vi "SonarsUpdate.vi"() -> ()   [LabVIEW 2016]
uses:
  <vilib>/Rock Robotics/WPI/Ultrasonic/WPI_UltrasonicRangeUnits.ctl
  <vilib>/Rock Robotics/WPI/Ultrasonic/WPI_SonarSRF04DigitalRefNum Registry Get.vi
  <vilib>/Rock Robotics/WPI/Ultrasonic/WPI_SonarSRF04DigitalGetRange.vi
  Globals/Globals.vi
  <vilib>/Rock Robotics/Network Tables/NT Write Number.vi
panel:
  in  "Sensor Droite Enable":bool
  in  "Sensor Gauche Enable":bool
  out "Waveform G":dbl(graph)
  out "Sensor Gauche":dbl
  out "Waveform  D":dbl(graph)
  out "Sensor Droite":dbl
  in  "Sensors Ping Duration (s)":sgl=1e-05
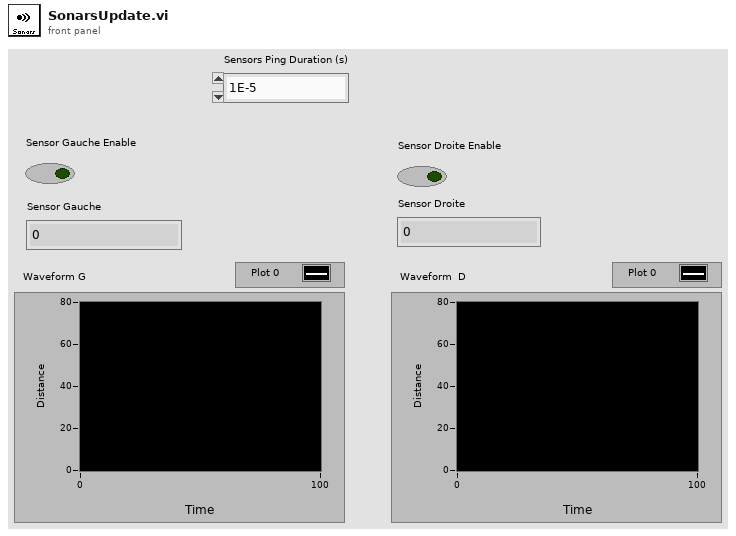
[diagram p1: front panel]
types:
  T1 = typedef "WPI_UltrasonicRangeUnits.ctl" = enum16{"inches", "mm"}
  T2 = typedef "WPI_UltrasonicDeviceRef.ctl" = cluster{"DevStatus":errorcluster, "Ping Channel":T3, "Echo Channel":T3, "CntIndex":T4}
  T3 = typedef "FPGA_DIOChannel.ctl" = enum8{"DIO 0", "DIO 1", "DIO 2", "DIO 3", "DIO 4", "DIO 5", "DIO 6", "DIO 7", "DIO 8", "DIO 9", "DIO MXP 0", "DIO MXP 1", "DIO MXP 2", "DIO MXP 3", "DIO MXP 4", "DIO MXP 5", "DIO MXP 6", "DIO MXP 7", "DIO MXP 8", "DIO MXP 9", "DIO MXP 10", "DIO MXP 11", "DIO MXP 12", "DIO MXP 13", "DIO MXP 14", "DIO MXP 15", "SPI Port CS1", "SPI Port CS2", "SPI Port CS3", "SPI Port MISO", "SPI Port MOSI", "Invalid"}
  T4 = typedef "FPGA_CounterCtrSystemIndex.ctl" = enum8{"Ctr 0", "Ctr 1", "Ctr 2", "Ctr 3", "Ctr 4", "Ctr 5", "Ctr 6", "Ctr 7", "Invalid"}
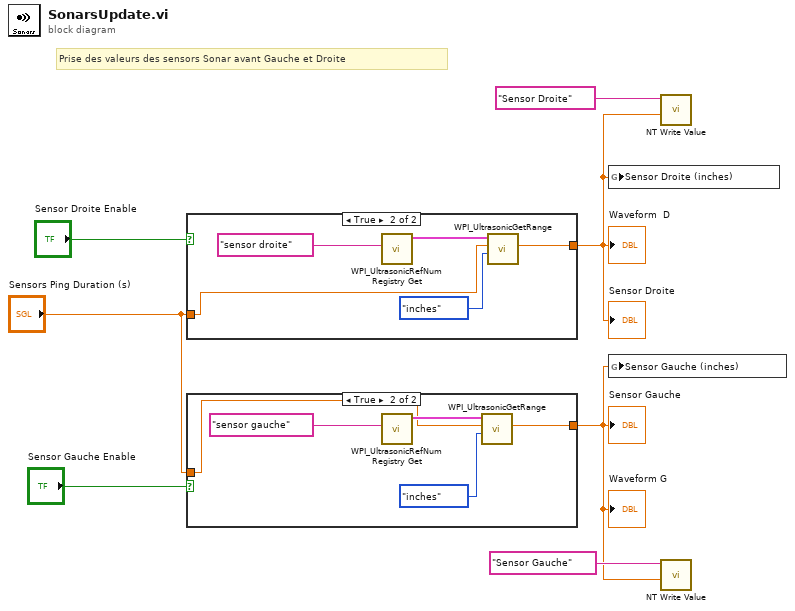
[diagram p0: block diagram]
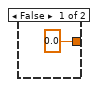
[diagram p2: hidden frame]
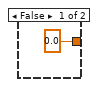
[diagram p3: hidden frame]
diagram:
  # "Prise des valeurs des sensors Sonar avant Gauche et Droite"
  n1 = case shown="True" "Sensor Droite Enable" {
    tunnel: "Sensors Ping Duration (s)" -> [_ w10]
    tunnel: [0.0 ("Distance") w9] -> w5
    frame False {
    }
    frame True {
      n2 = call-poly <vilib>:"WPI_UltrasonicRefNum Registry Get.vi"("refnum name"="sensor droite") -> ("SonarSRF04DevRef"=w13:T2)  [unwired: 9 in, 1 out]
      n3 = call-poly <vilib>:"WPI_UltrasonicGetRange.vi"("Range Units"=WPI_UltrasonicRangeUnits."inches", "ping time (s)"=w10, "SonarSRF04DevRef"=w13) -> ("Distance"=w9:dbl)  [unwired: 6 in, 2 out]
    }
  }
  "Sensor Droite" <- w5
  "Waveform  D" <- w5
  n4 = case shown="True" "Sensor Gauche Enable" {
    tunnel: "Sensors Ping Duration (s)" -> [_ w16]
    tunnel: [0.0 ("Distance") w15] -> w4
    frame False {
    }
    frame True {
      n5 = call-poly <vilib>:"WPI_UltrasonicRefNum Registry Get.vi"("refnum name"="sensor gauche") -> ("SonarSRF04DevRef"=w19:T2)  [unwired: 9 in, 1 out]
      n6 = call-poly <vilib>:"WPI_UltrasonicGetRange.vi"("Range Units"=WPI_UltrasonicRangeUnits."inches", "ping time (s)"=w16, "SonarSRF04DevRef"=w19) -> ("Distance"=w15:dbl)  [unwired: 6 in, 2 out]
    }
  }
  "Sensor Gauche" <- w4
  "Waveform G" <- w4
  n7 = global write "Globals.vi" "Sensor Droite (inches)"(w5) -> ()
  n8 = global write "Globals.vi" "Sensor Gauche (inches)"(w4) -> ()
  n9 = call-poly <vilib>:"NT Write Value.vi"("Numeric"=w5, "Name"="Sensor Droite") -> ()  [unwired: 9 in, 1 out]
  n10 = call-poly <vilib>:"NT Write Value.vi"("Numeric"=w4, "Name"="Sensor Gauche") -> ()  [unwired: 9 in, 1 out]
